vi "Tosca-Release IPC.vi"(7 "IPC":T1) -> (15 "error out":errorcluster)   [LabVIEW 2020]
uses:
  Tosca-IPC.ctl
  Classes/Parameters/Parameters.lvclass
  Digital Input VIs/Tosca-DI Queue Data.ctl
  Digital Input VIs/Tosca-Input Event.ctl
  Digital Input VIs/Tosca-Input Criterion.ctl
  epl-vi-lib/Utility VIs/Type Defs/Logic State.ctl
  Typedefs/Tosca-Accumulator.ctl
  Typedefs/Tosca-State AODO.ctl
  Typedefs/Tosca-AO Runtime.ctl
  Typedefs/Tosca-DO Runtime.ctl
  epl-vi-lib/Signal Synthesis VIs/4th Generation/Classes/SignalManager/SignalManager.lvclass
  Typedefs/Tosca-Synapse Start Data.ctl
  Tosca-Message.ctl
  Tosca-Message Action.ctl
  Typedefs/Tosca-Thread Type.ctl
  Imaging VIs/Tosca-2P-Notifier Data.ctl
  Typedefs/Tosca-MATLAB Queue Data.ctl
  Visual Stim VIs/Tosca-Grating.ctl
  Visual Stim VIs/Tosca-Grating Type.ctl
  Typedefs/Tosca-File IO Notification.ctl
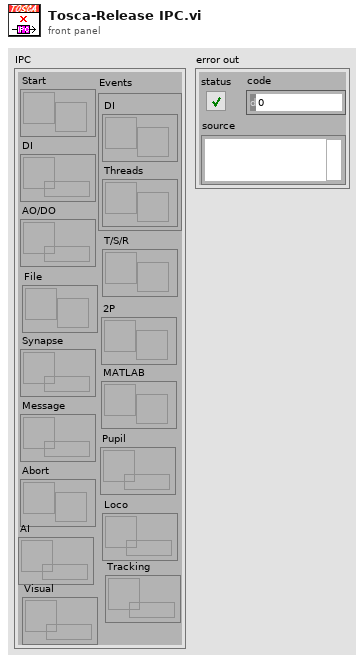
[diagram p1: front panel]
types:
  T1 = typedef "Tosca-IPC.ctl" = cluster{"Start":refnum<notifier>, "DI":refnum<queue>, "AO/DO":refnum<queue>, "Synapse":refnum<queue>, "Message":refnum<queue>, "Abort":refnum<notifier>, "Events":cluster{"DI":refnum<user-event>, "Threads ":refnum<user-event>}, "T/S/R":refnum<notifier>, "2P":refnum<notifier>, "MATLAB":refnum<notifier>, "Pupil":refnum<queue>, "Loco":refnum<queue>, "AI":refnum<queue>, "Tracking":refnum<queue>, "Visual":refnum<queue>, "File":refnum<notifier>}
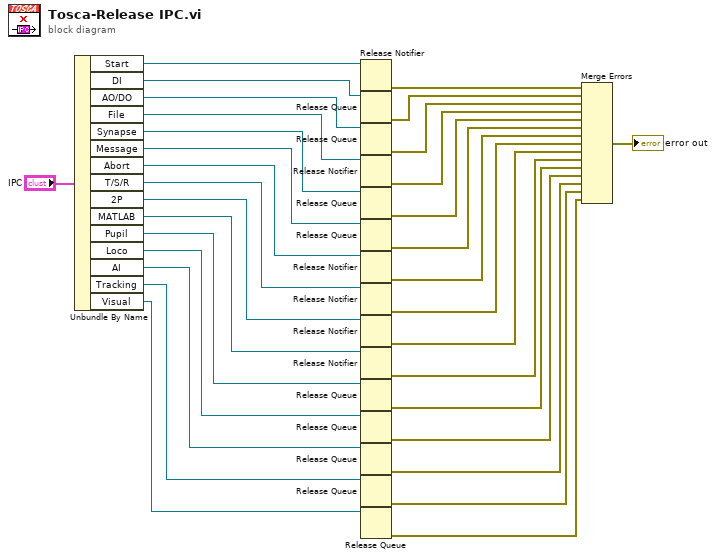
[diagram p0: block diagram]
diagram:
  n1 = Unbundle By Name("IPC") -> ("Start"=w26:refnum<notifier>, "DI"=w25:refnum<queue>, "AO/DO"=w24:refnum<queue>, "File"=w22:refnum<notifier>, "Synapse"=w23:refnum<queue>, "Message"=w20:refnum<queue>, "Abort"=w18:refnum<notifier>, "T/S/R"=w16:refnum<notifier>, "2P"=w14:refnum<notifier>, "MATLAB"=w12:refnum<notifier>, "Pupil"=w10:refnum<queue>, "Loco"=w8:refnum<queue>, "AI"=w6:refnum<queue>, "Tracking"=w4:refnum<queue>, "Visual"=w2:refnum<queue>)
  n2 = Release Notifier(notifier=w26) -> (error out=w32:errorcluster)  [unwired: 2 in, 2 out]
  n3 = Release Queue(queue=w25) -> (error out=w31:errorcluster)  [unwired: 2 in, 2 out]
  n4 = Release Queue(queue=w24) -> (error out=w30:errorcluster)  [unwired: 2 in, 2 out]
  n5 = Release Notifier(notifier=w22) -> (error out=w21:errorcluster)  [unwired: 2 in, 2 out]
  n6 = Release Queue(queue=w23) -> (error out=w29:errorcluster)  [unwired: 2 in, 2 out]
  n7 = Release Queue(queue=w20) -> (error out=w19:errorcluster)  [unwired: 2 in, 2 out]
  n8 = Release Notifier(notifier=w18) -> (error out=w17:errorcluster)  [unwired: 2 in, 2 out]
  n9 = Release Notifier(notifier=w16) -> (error out=w15:errorcluster)  [unwired: 2 in, 2 out]
  n10 = Release Notifier(notifier=w14) -> (error out=w13:errorcluster)  [unwired: 2 in, 2 out]
  n11 = Release Notifier(notifier=w12) -> (error out=w11:errorcluster)  [unwired: 2 in, 2 out]
  n12 = Release Queue(queue=w10) -> (error out=w9:errorcluster)  [unwired: 2 in, 2 out]
  n13 = Release Queue(queue=w8) -> (error out=w7:errorcluster)  [unwired: 2 in, 2 out]
  n14 = Release Queue(queue=w6) -> (error out=w5:errorcluster)  [unwired: 2 in, 2 out]
  n15 = Release Queue(queue=w4) -> (error out=w3:errorcluster)  [unwired: 2 in, 2 out]
  n16 = Release Queue(queue=w2) -> (error out=w1:errorcluster)  [unwired: 2 in, 2 out]
  n17 = Merge Errors(w32, w31, w30, w21, w29, w19, w17, w15, w13, w11, w9, w7, w5, w3, w1) -> (→"error out":errorcluster)
